vi "Clear Node Selection.vi"(8 "error in (no error)":errorcluster, 9 "New selection":i32=-1, 11 "FSM in":refnum<class "FSM.Graph.lvclass">) -> (0 "error out":errorcluster, 3 "FSM out":refnum<class "FSM.Graph.lvclass">)   [LabVIEW 2015, in "FSM.Graph.lvclass"]
uses:
  FSM.Graph.lvclass
  FSM.Graph.lvclass/FSM.Graph.ctl
  FSM.Node/FSM.Node.lvclass/FSM.Node.ctl
  FSM.Node/Write selected.vi
  FSM.Node/FSM.Node.lvclass
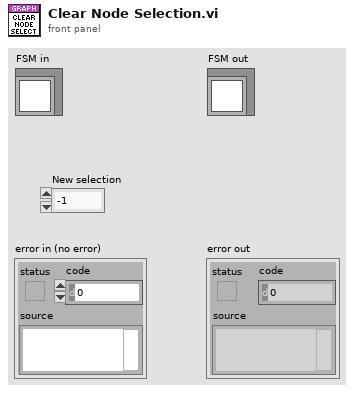
[diagram p1: front panel]
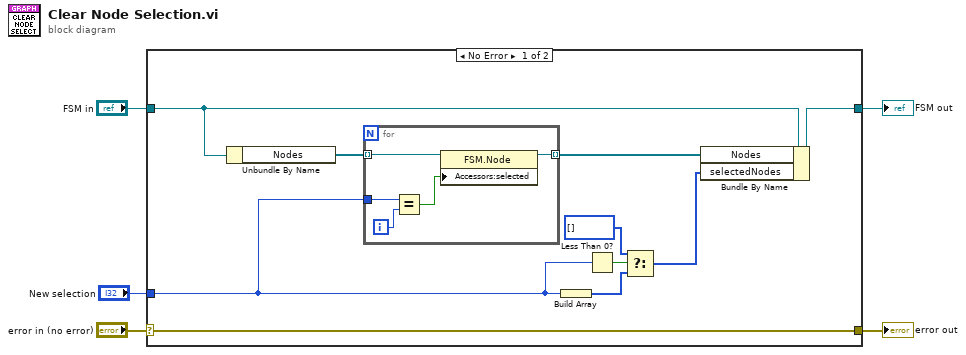
[diagram p0: block diagram]
diagram:
  n1 = case shown="No Error" "error in (no error)" {
    selector: "error in (no error)" -> [w15 w22]
    tunnel: [w15 w22] -> w4
    tunnel: [w12 w21] -> w2
    tunnel: "FSM in" -> [w14 w21]
    tunnel: "New selection" -> [w6 _]
    frame No Error {
      n2 = Unbundle By Name(w14) -> ("Nodes"=w13:refnum<class "FSM.Node.lvclass">[])
      n3 = for {
        tunnel: w13 -> [w20] mode=indexing
        tunnel: [w19] -> w11 mode=indexing
        tunnel: w6 -> [w18]
        i -> [w17]
        n4 = Equal?(x=w18, y=w17) -> (x = y?=w16:bool)
        n5 = property class="FSM.Node"(reference=w20, "Accessors:selected"=w16) -> (reference out=w19:refnum<class "FSM.Node.lvclass">)  [unwired: 1 in, 1 out]
      }
      n6 = Build Array(w6) -> (w7:i32[])
      n7 = Less Than 0?(x=w6) -> (x < 0?=w10:bool)
      n8 = Select(t=i32[] [] ("selectedNodes"), s=w10, f=w7) -> (s? t:f=w8:i32[])
      n9 = Bundle By Name(cluster=w14, "Nodes"=w11, "selectedNodes"=w8) -> (w12:refnum<class "FSM.Graph.lvclass">)
    }
    frame Error {
    }
  }
  "error out" <- w4
  "FSM out" <- w2
